vi "set property.vi"(8 "error in":errorcluster, 9 "propertynode_id":string, 10 "properties_iswrite":bool[](array[boolean]), 11 "property_ids":string[](array[string])) -> (0 "error out":errorcluster)   [LabVIEW 2020]
doc: "Sets the properties of a property-node. Set the property ids with property_ids string-array and their read/write state with properties_iswrite"
uses:
  G-AI Core/G-AI Core.lvlib
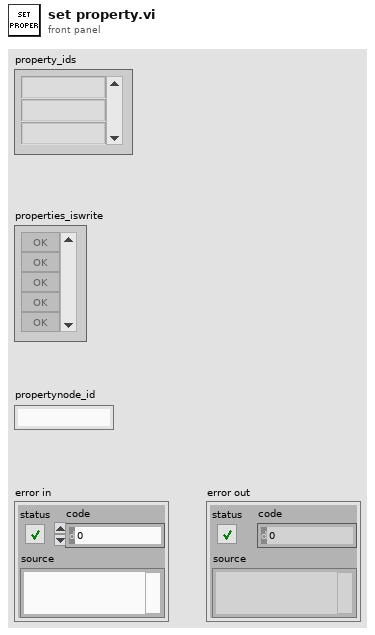
[diagram p1: front panel]
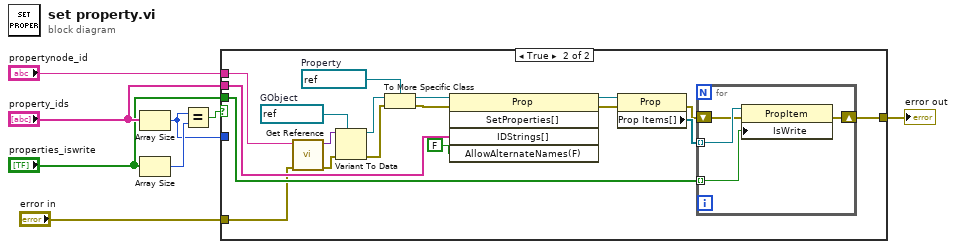
[diagram p0: block diagram]
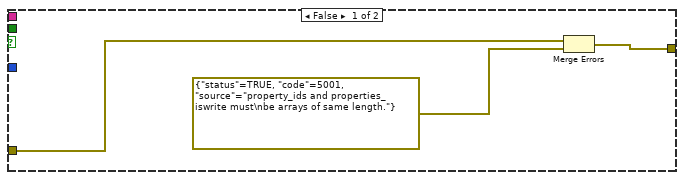
[diagram p2: hidden frame]
diagram:
  n1 = Array Size(array="property_ids") -> (size(s)=w5:i32)
  n2 = Array Size(array="properties_iswrite") -> (size(s)=w8:i32)
  n3 = Equal?(x=w5, y=w8) -> (x = y?=w6:bool)
  n4 = case shown="True" w6 {
    tunnel: [w10 w20] -> w7
    tunnel: w5 -> [_ _]
    tunnel: "property_ids" -> [_ w16]
    tunnel: "properties_iswrite" -> [_ w15]
    tunnel: "propertynode_id" -> [_ w14]
    tunnel: "error in" -> [w9 w12]
    frame False {
      n5 = Merge Errors(w9, errorcluster {"status"=TRUE, "code"=5001, "source"="property_ids and properties_iswrite must\nbe arrays of same length."} ("error out")) -> (w10:errorcluster)
    }
    frame True {
      w25 = refnum<vi> refnum  # Property
      w26 = refnum<vi> refnum  # GObject
      n6 = call "Get Reference.vi"("error in"=w12, "id"=w14) -> ("error out"=w29:errorcluster, "reference"=w28:variant)  [unwired: 8 in]
      n7 = Variant To Data(error in=w29, type=w26, Variant=w28) -> (data=w24:refnum<vi>, error out=w27:errorcluster)
      n8 = To More Specific Class(target class=w25, reference=w24, error in=w27) -> (specific class reference=w18:refnum<vi>, error out=w23:errorcluster)
      n9 = invoke class="Prop" method="SetProperties[]"(reference=w18, error in=w23, "IDStrings[]"=w16, "AllowAlternateNames(F)"=FALSE ("Allow Alternate Names? (F)")) -> (reference out=w17:refnum<vi>, error out=w19:errorcluster)  [unwired: 1 in, 3 out]
      n10 = property class="Prop"(reference=w17, error in=w19) -> (error out=w21:errorcluster, "Prop Items[]"=w22:refnum<vi>[])  [unwired: 1 out]
      n11 = for {
        tunnel: w22 -> [w33] mode=indexing
        shift-right: [w31] -> w20
        shift-left: w21 -> [w32]
        tunnel: w15 -> [w30] mode=indexing
        n12 = property class="PropItem"(reference=w33, error in=w32, "IsWrite"=w30) -> (error out=w31:errorcluster)  [unwired: 1 out]
      }
    }
  }
  "error out" <- w7
